vi "Scan Engine Slot Page.vi"(8 "error in (no error)":errorcluster, 11 "Node Ptr":T2 format="%.0x") -> (0 "error out":errorcluster)   [LabVIEW 2016, in "Scan Engine Custom Device.lvlib"]
uses:
  Scan Engine Custom Device.lvlib
  <vilib>/NI Veristand/Custom Device API/Custom Device API.lvlib
  Modules.lvlibp/RSI Module/SubPanel Command.ctl
  Globals/Scan Engine GUIDs.vi
  <vilib>/NI Veristand/Custom Device API/Custom Device Item Ref.ctl
  Modules.lvlibp/RSI Module/Module Models.ctl
panel:
  out "Slot #":u32
  in  "Module":T1
  in  "Header":cluster{"Section Name":string}={"Section Name"="Slot Settings"}
  in  "Description":string
  out "Name":string
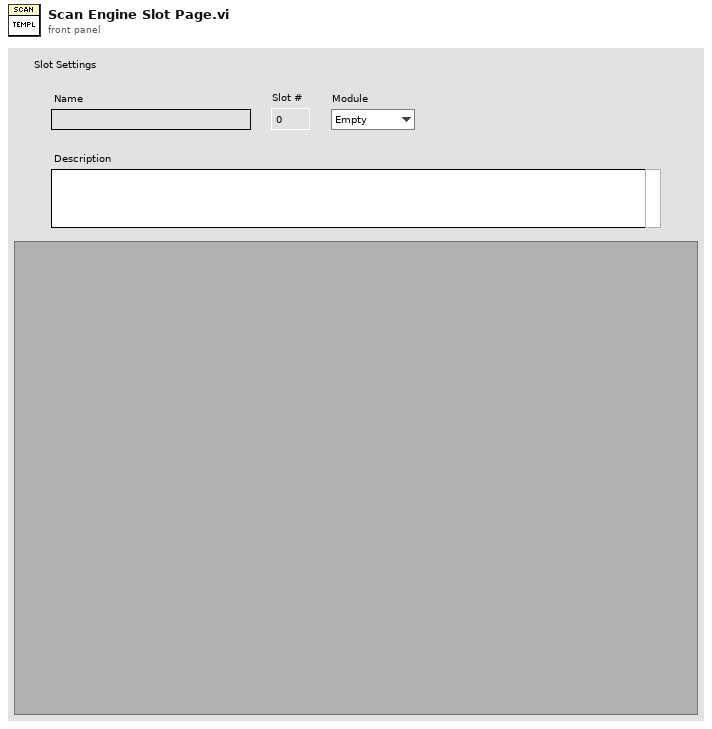
[diagram p1: front panel]
types:
  T1 = typedef "Modules.lvlibp/RSI Module.lvclass/Module Models.ctl" = enum16{"Empty", "NI 9201", "NI 9203", "NI 9205", "NI 9206", "NI 9207", "NI 9208", "NI 9211", "NI 9213", "NI 9214", "NI 9215", "NI 9217", "NI 9219", "NI 9221", "NI 9225", "NI 9227", "NI 9229", "NI 9233", "NI 9234", "NI 9235", "NI 9236", "NI 9237", "NI 9239", "NI 9263", "NI 9264", "NI 9265", "NI 9269", "NI 9375", "NI 9401", "NI 9402", "NI 9403", "NI 9411", "NI 9421", "NI 9422", "NI 9423", "NI 9425", "NI 9426", "NI 9435", "NI 9472", "NI 9474", "NI 9475", "NI 9476", "NI 9477", "NI 9478", "NI 9481", "NI 9482", "NI 9485"}
  T2 = typedef "Custom Device API.lvlib/Custom Device Item Ref.ctl" = u64
  T3 = enum8{"Enabled", "Disabled", "Disabled and Grayed Out"}
  T4 = typedef "Custom Device API.lvlib/Custom Device Item Info.ctl" = cluster{"Name":string, "Is Channel":bool, "GUID":string, "Is Waveform":bool}
  T5 = typedef "Modules.lvlibp/RSI Module.lvclass/SubPanel Command.ctl" = enum16{"Stop"}
  T6 = typedef "Custom Device API.lvlib/Custom Device Commands.ctl" = enum16{"Default", "Item renamed", "Shutdown", "Dynamic button pressed"}
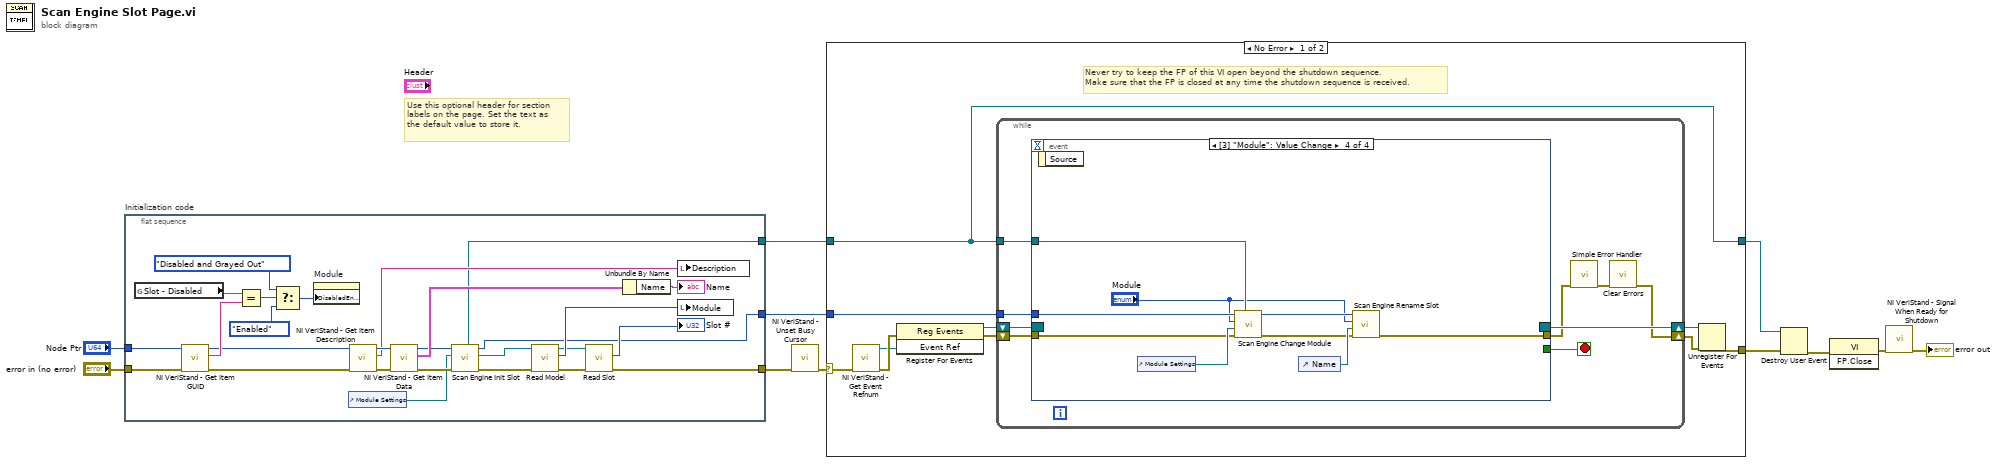
[diagram p0: block diagram]
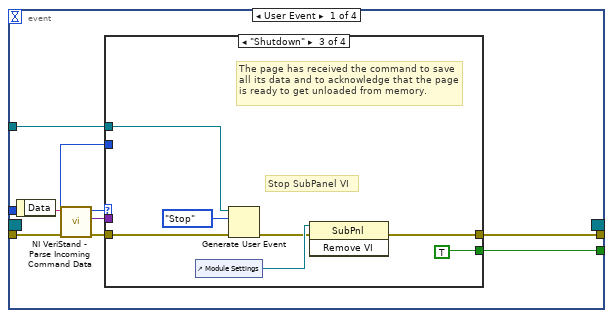
[diagram p2: hidden frame]
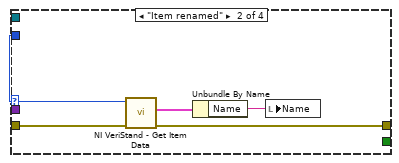
[diagram p4: hidden frame]
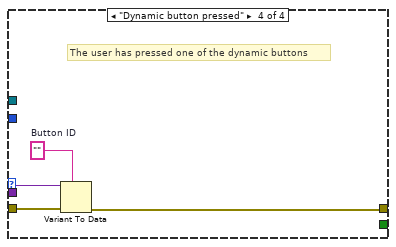
[diagram p5: hidden frame]
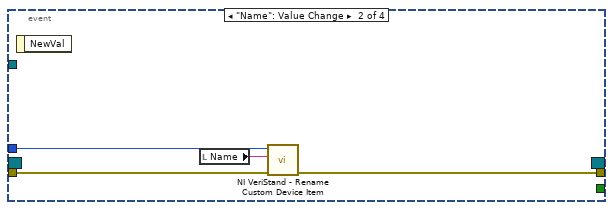
[diagram p6: hidden frame]
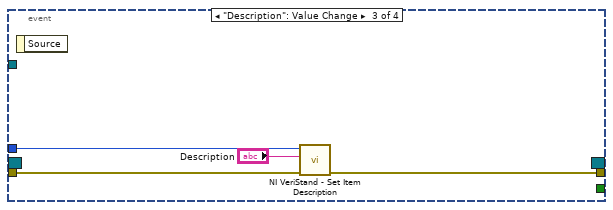
[diagram p7: hidden frame]
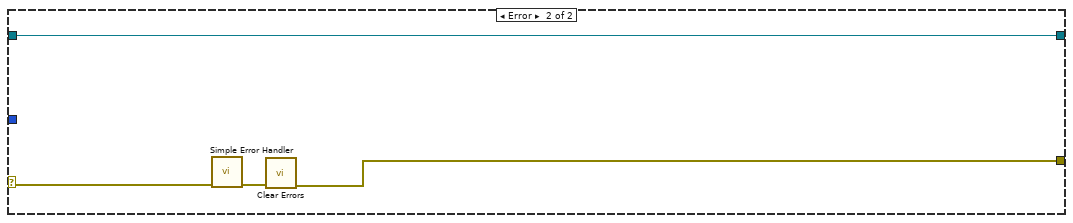
[diagram p8: hidden frame]
diagram:
  # "Use this optional header for section labels on the page. Set the text as the default value to store it."
  n1 = flat-sequence "Initialization code" {
    tunnel: "error in (no error)" -> [w20]
    tunnel: "Node Ptr" -> [w21]
    tunnel: [w22] -> w8
    tunnel: [w24] -> w5
    tunnel: [w26] -> w4
    frame #0 {
      n2 = global read "Scan Engine GUIDs.vi" "Slot - Disabled"() -> (w19:string)
      n3 = call <vilib>:"NI VeriStand - Get Item GUID.vi"("error in (no error)"=w20, "Item Ref in"=w21) -> ("error out"=w16:errorcluster, "GUID"=w18:string, "Item Ref out"=w17:T2)  [unwired: 7 in]
      n4 = Equal?(x=w19, y=w18) -> (x = y?=w15:bool)
      n5 = Select(t=T3."Disabled and Grayed Out" ("Disabled"), s=w15, f=T3."Enabled" ("Disabled")) -> (s? t:f=w12:T3)
      n6 = property on="Module" class="Enum (strict)"("DisabledEnum"=w12) -> ()  [unwired: 2 in, 2 out]
      n7 = control-ref of="Module Settings"() -> (w27:refnum<vi>)
      n8 = call <vilib>:"NI VeriStand - Get Item Description.vi"("error in (no error)"=w16, "Item Ref in"=w17) -> ("error out"=w36:errorcluster, "Description"=w37:string, "Item Ref out"=w38:T2)  [unwired: 7 out]
      n9 = call <vilib>:"NI VeriStand - Get Item Data.vi"("error in (no error)"=w36, "Item Ref in"=w38) -> ("error out"=w29:errorcluster, "Item Info"=w35:T4, "Item Ref out"=w28:T2)  [unwired: 7 out]
      n10 = call "Scan Engine Init Slot.vi"("error in (no error)"=w29, "SubPanel Ref"=w27, "Node Ptr In"=w28) -> ("error out"=w23:errorcluster, "RSI Module"=w25:refnum<class "RSI Module.lvclass">, "Node Ptr Out"=w24:T2, "SubPanel Command"=w26:refnum<user-event>)  [unwired: 5 in]
      n11 = call "Read Model.vi"("error in (no error)"=w23, "RSI Module in"=w25) -> ("error out"=w31:errorcluster, "Model"=w33:T1, "RSI Module out"=w32:refnum<class "RSI Module.lvclass">)  [unwired: 7 in]
      n12 = call "Read Slot.vi"("error in (no error)"=w31, "RSI Module in"=w32) -> ("error out"=w22:errorcluster, "Slot"=→"Slot #":u32)  [unwired: 7 in, 1 out]
      n13 = Unbundle By Name(w35) -> ("Name"=→"Name":string)
      n14 = local write "Description"(w37) -> ()
      n15 = local write "Module"(w33) -> ()
    }
  }
  n16 = call <vilib>:"NI VeriStand - Unset Busy Cursor.vi"("error in (no error)"=w8) -> ("error out"=w7:errorcluster)  [unwired: 10 out]
  n17 = case shown="No Error" w7 {
    selector: w7 -> [w40 w104]
    tunnel: [w45 w102] -> w2
    tunnel: w5 -> [w41 _]
    tunnel: w4 -> [w39 w101]
    tunnel: [w39 w101] -> w3
    frame No Error {
      # "Never try to keep the FP of this VI open beyond the shutdown sequence.\nMake sure that the FP is closed at any time the shutdown sequence is received."
      n18 = call <vilib>:"NI VeriStand - Get Event Refnum.vi"("error in (no error)"=w40) -> ("error out"=w48:errorcluster, "Event Ref"=w44:refnum<user-event>)  [unwired: 9 out]
      n19 = register-events(error in=w48, w44) -> (reference out=w42:refnum<event-registration>, error out=w43:errorcluster)  [unwired: 1 in]
      n20 = while {
        tunnel: w41 -> [w53]
        shift-right: [w50] -> w46
        shift-left: w43 -> [w56]
        shift-right: [w57] -> w47
        shift-left: w42 -> [w55]
        tunnel: w39 -> [w49]
        stop <- w54 stop-if-true
        n21 = event shown="[3] \"Module\": Value Change" {
          selector: w55 -> [_ _ _ _]
          dyn-events: [_ _ _ _] -> w57
          timeout: _ -> [_ _ _ _]
          tunnel: w56 -> [w66 w87 w90 w97]
          tunnel: [w62 _ _ _] -> w54
          tunnel: [w61 w86 w89 w92] -> w52
          tunnel: w53 -> [w60 w85 w91 w96]
          tunnel: w49 -> [w58 _ _ w98]
          event User Event {
            n22 = event-data() -> ("Data"=w65:string)  [unwired: 1 out]
            n23 = call <vilib>:"NI VeriStand - Parse Incoming Command Data.vi"("error in (no error)"=w66, "Incoming data"=w65) -> ("error out"=w64:errorcluster, "Outgoing data"=w59:variant, "Action"=w63:T6)  [unwired: 7 out]
            n24 = case shown="\"Shutdown\"" w63 {
              tunnel: w64 -> [w67 w72 w76 w83]
              tunnel: [_ _ TRUE _] -> w62
              tunnel: [w67 w69 w73 w80] -> w61
              tunnel: w60 -> [_ w71 _ _]
              tunnel: w59 -> [_ _ _ w82]
              tunnel: w58 -> [_ _ w78 _]
              frame "Default", Default {
              }
              frame "Item renamed" {
                n25 = call <vilib>:"NI VeriStand - Get Item Data.vi"("error in (no error)"=w72, "Item Ref in"=w71) -> ("error out"=w69:errorcluster, "Item Info"=w70:T4)  [unwired: 8 out]
                n26 = Unbundle By Name(w70) -> ("Name"=w68:string)
                n27 = local write "Name"(w68) -> ()
              }
              frame "Shutdown" {
                # "Stop SubPanel VI"
                # "The page has received the command to save all its data and to acknowledge that the page is ready to get unloaded from memory."
                n28 = control-ref of="Module Settings"() -> (w75:refnum<vi>)
                n29 = Generate User Event(user event=w78, event data cluster=SubPanel_Command."Stop" ("event data"), error in=w76) -> (error out=w74:errorcluster)  [unwired: 1 in, 1 out]
                n30 = invoke class="SubPnl" method="Remove VI"(reference=w75, error in=w74) -> (error out=w73:errorcluster)  [unwired: 1 in, 2 out]
              }
              frame "Dynamic button pressed" {
                w81 = ""  # Button ID
                # "The user has pressed one of the dynamic buttons"
                n31 = Variant To Data(error in=w83, type=w81, Variant=w82) -> (error out=w80:errorcluster)  [unwired: 1 out]
              }
            }
          }
          event "Name": Value Change {
            n32 = event-data() -> ()  [unwired: 2 out]
            n33 = local read "Name"() -> (w84:string)
            n34 = call <vilib>:"NI VeriStand - Rename Custom Device Item.vi"("error in (no error)"=w87, "New Name"=w84, "Item Ref in"=w85) -> ("error out"=w86:errorcluster)  [unwired: 1 in, 7 out]
          }
          event "Description": Value Change {
            n35 = event-data() -> ()  [unwired: 2 out]
            n36 = call <vilib>:"NI VeriStand - Set Item Description.vi"("error in (no error)"=w90, "Description"="Description", "Item Ref in"=w91) -> ("error out"=w89:errorcluster)  [unwired: 8 out]
          }
          event Value Change {
            n37 = event-data() -> ()  [unwired: 2 out]
            n38 = control-ref of="Module Settings"() -> (w99:refnum<vi>)
            n39 = call "Scan Engine Change Module.vi"("SubPanel Event"=w98, "error in (no error)"=w97, "SubPanel Ref"=w99, "Module Model"="Module", "Node Ptr In"=w96) -> ("error out"=w93:errorcluster, "Node Ptr Out"=w95:T2)  [unwired: 5 in]
            n40 = control-ref of="Name"() -> (w100:refnum<vi>)
            n41 = call "Scan Engine Rename Slot.vi"("error in (no error)"=w93, "Name reference"=w100, "Module Model"="Module", "Node Ptr In"=w95) -> ("error out"=w92:errorcluster)  [unwired: 6 in, 1 out]
          }
        }
        n42 = call <vilib>:"Simple Error Handler.vi"("error in (no error)"=w52) -> ("error out"=w51:errorcluster)  [unwired: 1 in, 7 out]
        n43 = call <vilib>:"Clear Errors.vi"("error in (no error)"=w51) -> ("error out"=w50:errorcluster)  [unwired: 1 in, 5 out]
      }
      n44 = Unregister For Events(event registration refnum=w47, error in=w46) -> (error out=w45:errorcluster)
    }
    frame Error {
      n45 = call <vilib>:"Simple Error Handler.vi"("error in (no error)"=w104) -> ("error out"=w103:errorcluster)  [unwired: 1 in, 7 out]
      n46 = call <vilib>:"Clear Errors.vi"("error in (no error)"=w103) -> ("error out"=w102:errorcluster)  [unwired: 1 in, 5 out]
    }
  }
  n47 = Destroy User Event(user event=w3, error in=w2) -> (error out=w1:errorcluster)
  n48 = invoke class="VI" method="FP.Close"(error in=w1) -> (error out=w11:errorcluster)  [unwired: 2 in, 2 out]
  n49 = call <vilib>:"NI VeriStand - Signal When Ready for Shutdown.vi"("error in (no error)"=w11) -> ("error out"=→"error out":errorcluster)  [unwired: 10 out]
